vi "Remove.vi"(8 "error in (no error)":errorcluster, 10 "Test to Remove":string, 11 "LUnit Test Suite In":refnum<class "LUnit Test Suite.lvclass">) -> (0 "error out":errorcluster, 3 "LUnit Test Suite Out":refnum<class "LUnit Test Suite.lvclass">)   [LabVIEW 2020, in "LUnit Test Suite.lvclass"]
doc: "Remove a test by name from the test suite."
uses:
  LUnit Test Suite.lvclass
  C:/git/astemes-lunit/source/Core/Runnable/Runnable.lvclass
  LUnit Test Suite.lvclass/LUnit Test Suite.ctl
  Runnable/Runnable.lvclass
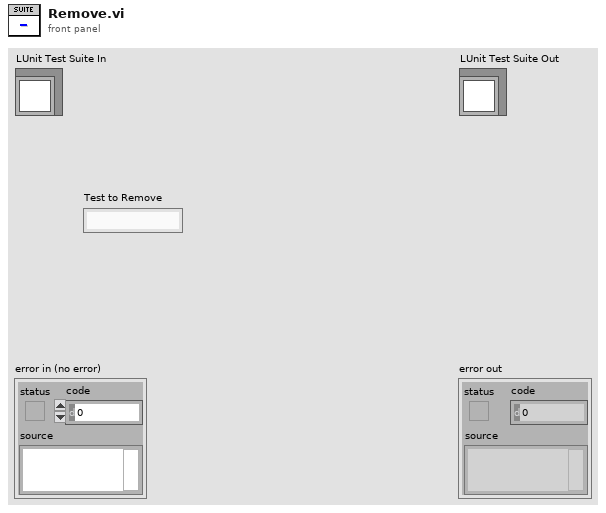
[diagram p1: front panel]
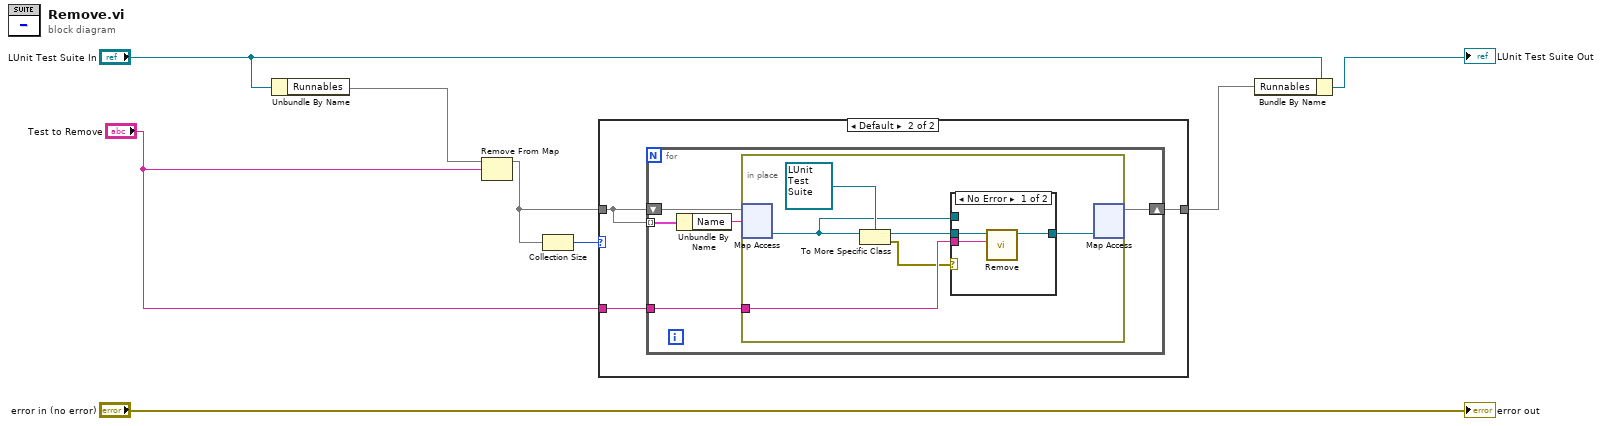
[diagram p0: block diagram]
diagram:
  n1 = Unbundle By Name("LUnit Test Suite In") -> ("Runnables"=w4:map{string, refnum<class "Runnable.lvclass">})
  n2 = Remove From Map(10:"Test to Remove", 11:w4) -> (3:w2:map{string, refnum<class "Runnable.lvclass">})  [unwired: 2 out]
  n3 = Collection Size(1:w2) -> (0:w1:i32)
  n4 = case shown="Default" w1 {
    tunnel: "Test to Remove" -> [_ w12]
    tunnel: [w9 w11] -> w3
    tunnel: w2 -> [w9 w10]
    frame 0 {
    }
    frame Default {
      n5 = for {
        tunnel: w10 -> [w16] mode=indexing
        shift-right: [w13] -> w11
        shift-left: w10 -> [w17]
        tunnel: w12 -> [w14]
        n6 = Unbundle By Name(w16) -> ("Name"=w15:string)
        n7 = in-place {
          in-place-border: w14 -> [w22]
          n8 = in-place-map #1(w17, w15) -> (w18:refnum<class "Runnable.lvclass">)  [unwired: 1 in, 1 out]
          n9 = To More Specific Class(target class=refnum<class "LUnit Test Suite.lvclass"> refnum ("LUnit Test Suite.lvclass"), reference=w18) -> (specific class reference=w19:refnum<class "LUnit Test Suite.lvclass">, error out=w20:errorcluster)  [unwired: 1 in]
          n10 = case shown="No Error" w20 {
            tunnel: w19 -> [w26 _]
            tunnel: w22 -> [w25 _]
            tunnel: [w24 w27] -> w21
            tunnel: w18 -> [_ w27]
            frame No Error {
              n11 = call "Remove.vi"("Test to Remove"=w25, "LUnit Test Suite In"=w26) -> ("LUnit Test Suite Out"=w24:refnum<class "LUnit Test Suite.lvclass">)  [unwired: 8 in, 1 out]
            }
            frame Error {
            }
          }
          n12 = in-place-map #1(w21) -> (w13:map{string, refnum<class "Runnable.lvclass">})  [unwired: 1 in, 2 out]
        }
      }
    }
  }
  n13 = Bundle By Name(cluster="LUnit Test Suite In", "Runnables"=w3) -> (→"LUnit Test Suite Out":refnum<class "LUnit Test Suite.lvclass">)
  "error out" <- "error in (no error)"
